vi "Read Publication Received Event.vi"(8 "error in (no error)":errorcluster, 11 "SubscriptionDetails JSON in":refnum<class "SubscriptionDetails JSON.lvclass">) -> (0 "error out":errorcluster, 2 "Publication Received Event":refnum<user-event>, 3 "SubscriptionDetails JSON out":refnum<class "SubscriptionDetails JSON.lvclass">)   [LabVIEW 2020, in "wamplv.lvlib" / "SubscriptionDetails JSON.lvclass"]
uses:
  SubscriptionDetails JSON.lvclass
  SubscriptionDetails JSON.lvclass/SubscriptionDetails JSON.ctl
  WAMP Client/Private/TypeDef/EVENT payload (JSON).ctl
  wamplv.lvlib
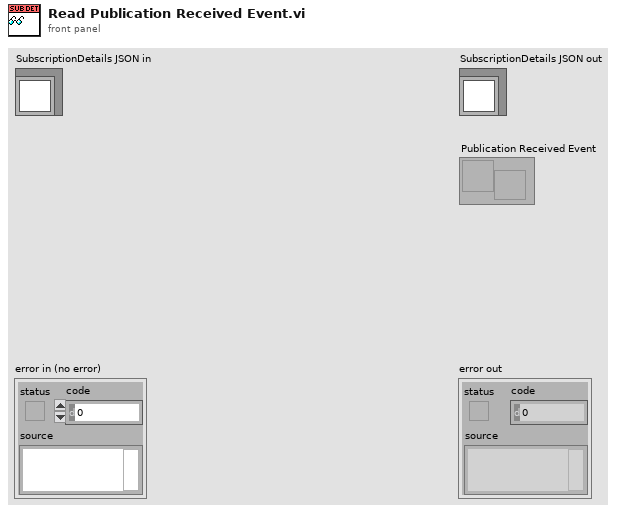
[diagram p1: front panel]
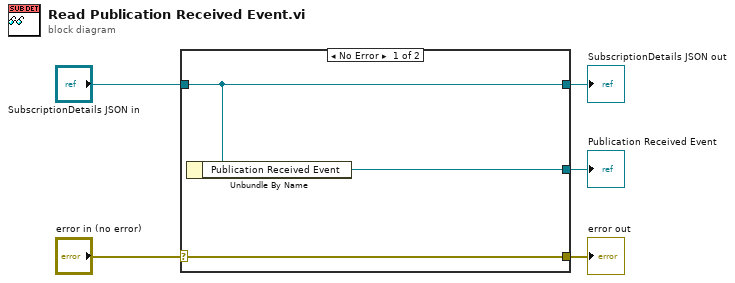
[diagram p0: block diagram]
diagram:
  n1 = case shown="No Error" "error in (no error)" {
    selector: "error in (no error)" -> [w8 w9]
    tunnel: [w8 w9] -> w4
    tunnel: [w7 w10] -> w2
    tunnel: "SubscriptionDetails JSON in" -> [w7 w10]
    tunnel: [w6 _] -> w1
    frame No Error {
      n2 = Unbundle By Name(w7) -> ("Publication Received Event"=w6:refnum<user-event>)
    }
    frame Error {
    }
  }
  "error out" <- w4
  "SubscriptionDetails JSON out" <- w2
  "Publication Received Event" <- w1
